vi "create.vi"(6 "Default Headers ([JSON])":T1[](array[typedef])=[{"header"="Content-Type", "value"="application/json"}], 8 "error in":errorcluster, 11 "Base URL":string) -> (0 "error out":errorcluster, 3 "reqwest":refnum<class "reqwest.lvclass">)   [LabVIEW 2020, in "reqwest.lvclass"]
uses:
  reqwest.lvclass
  header.ctl
  private_data.ctl
  reqwest.lvclass/reqwest.ctl
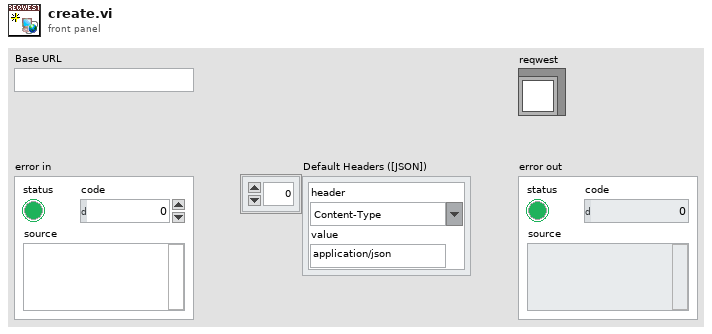
[diagram p1: front panel]
types:
  T1 = typedef "reqwest.lvclass/header.ctl" = cluster{"header":string, "value":string}
  T2 = typedef "reqwest.lvclass/private_data.ctl" = cluster{"Default Headers ([JSON])":T1[], "Base URL":string, "Authentication":cluster{"Username":string, "Password":string}}
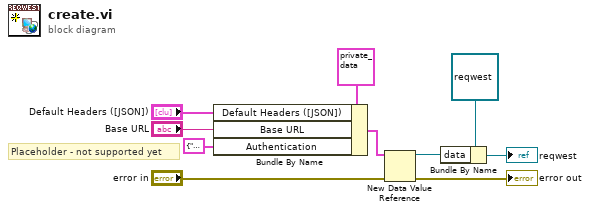
[diagram p0: block diagram]
diagram:
  # "Placeholder - not supported yet"
  n1 = Bundle By Name(cluster=T2 {"Default Headers ([JSON])"=[{"header"="Content-Type", "value"="application/json"}], "Base URL"="", "Authentication"={"Username"="", "Password"=""}} ("private data"), "Default Headers ([JSON])"="Default Headers ([JSON])", "Base URL"="Base URL", "Authentication"=cluster{"Username":string, "Password":string} {"Username"="", "Password"=""}) -> (w9:T2)
  n2 = New Data Value Reference(data value=w9, error in="error in") -> (data value reference=w7:refnum<data-value>, error out=→"error out":errorcluster)
  n3 = Bundle By Name(cluster=refnum<class "reqwest.lvclass"> refnum ("reqwest.lvclass"), "data"=w7) -> (→"reqwest":refnum<class "reqwest.lvclass">)
